vi "roboRIO v1.0 Close Encoder.vi"(8 "error in (no error)":errorcluster, 10 "Encoder Channel":T1, 11 "myRIO Ref In":T2) -> (0 "error out":errorcluster)   [LabVIEW 2021]
uses:
  <vilib>/myRIO/Common/Instrument Driver Framework/Utilities/typedefs/myRIO v1.0 Reference.ctl
  <vilib>/myRIO/Common/Instrument Driver Framework/Utilities/typedefs/Generic FPGA Reference.ctl
  <vilib>/myRIO/Common/Instrument Driver Framework/myRIO v1.0/Encoder/typedefs/Encoder Channels Enum.ctl
  <vilib>/myRIO/Common/Instrument Driver Framework/roboRIO v1.0/Resource Manager/vis/roboRIO v1.0 Unreserve Channel List.vi
  <vilib>/myRIO/Common/Instrument Driver Framework/roboRIO v1.0/Encoder/vis/roboRIO v1.0 Build MUX Configuration Encoder.vi
  <vilib>/myRIO/Common/Instrument Driver Framework/roboRIO v1.0/Resource Manager/vis/roboRIO v1.0 Unreserve Channel.vi
  <vilib>/myRIO/Common/Instrument Driver Framework/roboRIO v1.0/Resource Manager/vis/roboRIO v1.0 Create Configuration List.vi
  <vilib>/myRIO/Common/Instrument Driver Framework/roboRIO v1.0/Resource Manager/vis/roboRIO v1.0 Build Mutex Name.vi
  <vilib>/myRIO/Common/Instrument Driver Framework/roboRIO v1.0/Resource Manager/vis/roboRIO v1.0 Configure IO.vi
  <vilib>/myRIO/Common/Instrument Driver Framework/Utilities/vis/Configuration Manager.vi
  <vilib>/myRIO/Common/Instrument Driver Framework/Utilities/vis/IO Manager.vi
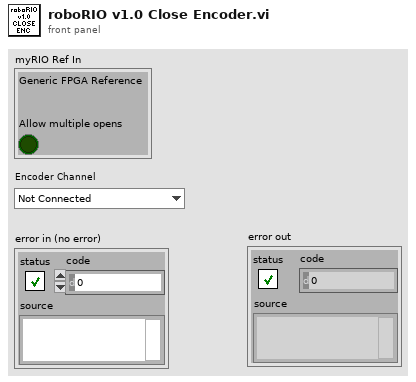
[diagram p1: front panel]
types:
  T1 = typedef "Encoder Channels Enum.ctl" = enum16{"Not Connected", "C/ENC0", "C/ENC1", "A/ENC", "A/ENC0", "A/ENC1", "A/ENC2", "A/ENC3", "A/ENC4", "A/ENC5", "A/ENC6", "A/ENC7", "A/ENC8", "A/ENC9", "B/ENC", "B/ENC0", "B/ENC1", "B/ENC2", "B/ENC3", "B/ENC4", "B/ENC5", "B/ENC6", "B/ENC7", "B/ENC8", "B/ENC9", "DIO/ENC0", "DIO/ENC1", "DIO/ENC2", "DIO/ENC3", "DIO/ENC4"}
  T2 = typedef "myRIO v1.0 Reference.ctl" = cluster{"Generic FPGA Reference":T3, "Allow multiple opens":bool}
  T3 = typedef "Generic FPGA Reference.ctl" = refnum<k20>
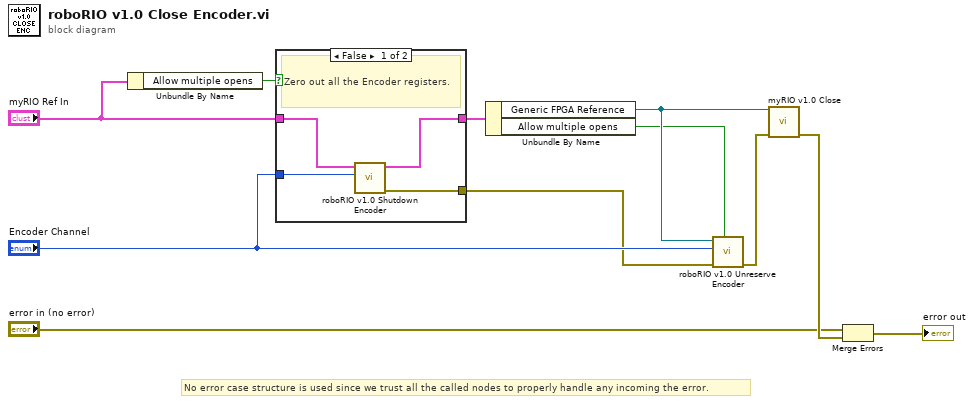
[diagram p0: block diagram]
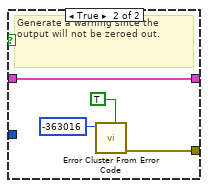
[diagram p2: hidden frame]
diagram:
  # "No error case structure is used since we trust all the called nodes to properly handle any incoming the error."
  n1 = Unbundle By Name("myRIO Ref In") -> ("Allow multiple opens"=w1:bool)
  n2 = case shown="False" w1 {
    tunnel: "myRIO Ref In" -> [w15 w19]
    tunnel: [w14 w19] -> w5
    tunnel: "Encoder Channel" -> [w13 _]
    tunnel: [w12 w16] -> w3
    frame False {
      # "Zero out all the Encoder registers."
      n3 = call <vilib>:"roboRIO v1.0 Shutdown Encoder.vi"("Channel"=w13, "myRIO Ref In"=w15) -> ("error out"=w12:errorcluster, "myRIO Ref Out"=w14:T2)  [unwired: 8 in]
    }
    frame True {
      # "Generate a warning since the output will not be zeroed out."
      n4 = call <vilib>:"Error Cluster From Error Code.vi"("is warning? (False)"=TRUE, "error code (0)"=-363016) -> ("error out"=w16:errorcluster)  [unwired: 7 in]
    }
  }
  n5 = Unbundle By Name(w5) -> ("Generic FPGA Reference"=w9:T3, "Allow multiple opens"=w8:bool)
  n6 = call <vilib>:"roboRIO v1.0 Unreserve Encoder.vi"("Allow multiple opens?"=w8, "error in (no error)"=w3, "Encoder Channel"="Encoder Channel", "myRIO FPGA Ref Out"=w9) -> ("error out"=w11:errorcluster)  [unwired: 7 in]
  n7 = call <vilib>:"myRIO v1.0 Close.vi"("error in (no error)"=w11, "myRIO FPGA Ref In"=w9) -> ("error out"=w10:errorcluster)  [unwired: 9 in]
  n8 = Merge Errors("error in (no error)", w10) -> (→"error out":errorcluster)
